vi "NXT_HINDBRAIN Battery Voltage To String.vi"(1 "_batteryVoltage":i32) -> (0 "String":string)   [LabVIEW 2012, in "Tugboat.lvrbt"]
uses:
  Tugboat.lvrbt
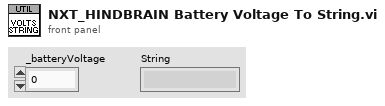
[diagram p1: front panel]
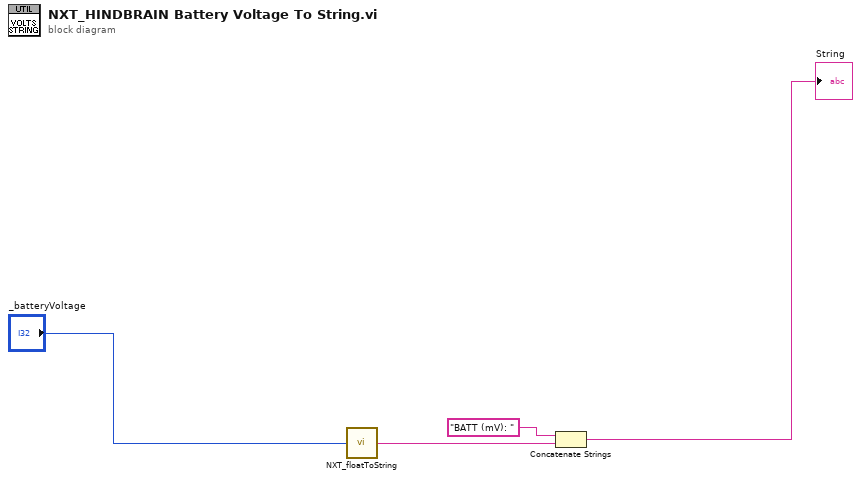
[diagram p0: block diagram]
diagram:
  n1 = call <vilib>:"NXT_floatToString.vi"("number"="_batteryVoltage") -> ("string"=w2:string)
  n2 = Concatenate Strings("BATT (mV): " ("string"), w2) -> (→"String":string)
